vi "CodeKeithley.vi"(11 "SweepInfo":T1={"Current Range"=1e-10, "Source Measure Unit Channel (0: Channel A)"=0, "Waveform"={"t0"=timestamp(0 s since 1904-01-01), "dt"=1.0, "Y"=[]}, "VISA resource name"="", "CodeText"=""}) -> (0 "error out":errorcluster)   [LabVIEW 2020]
uses:
  Keithley 2600 Series/Keithley 2600 Series.lvlib
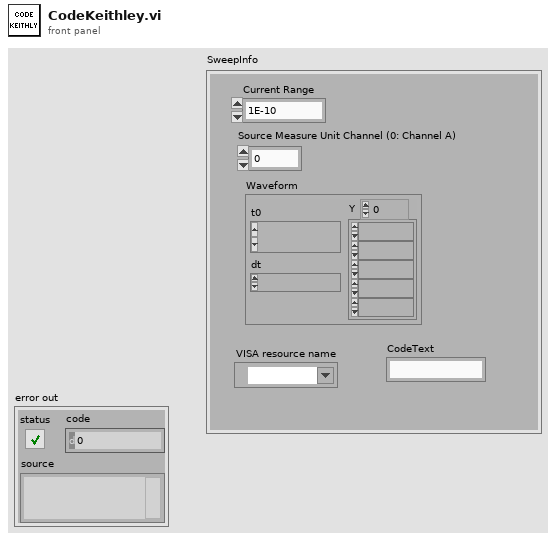
[diagram p1: front panel]
types:
  T1 = cluster{"Current Range":dbl, "Source Measure Unit Channel (0: Channel A)":i32, "Waveform":waveform(dbl), "VISA resource name":refnum<visa-resource-name>, "CodeText":string}
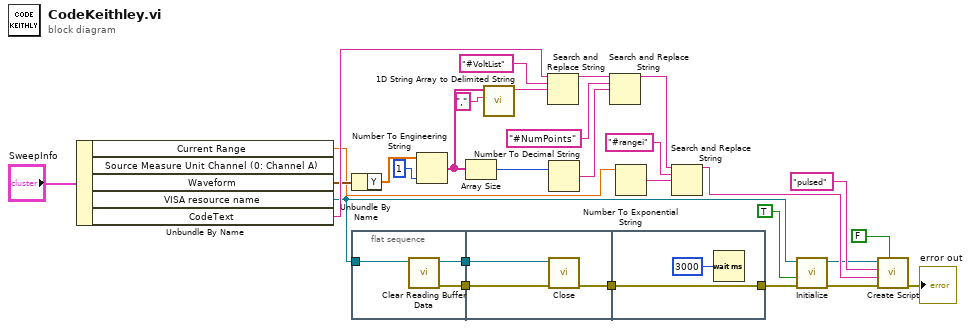
[diagram p0: block diagram]
diagram:
  n1 = Unbundle By Name("SweepInfo") -> ("Current Range"=w6:dbl, "Waveform"=w8:waveform(dbl), "VISA resource name"=w5:refnum<visa-resource-name>, "CodeText"=w9:string)  [unwired: 1 out]
  n2 = Unbundle By Name(w8) -> ("Y"=w20:dbl[])
  n3 = flat-sequence {
    tunnel: w5 -> [w32]
    tunnel: [w31] -> w4
    tunnel: [w30] -> w3
    tunnel: w4 -> [w35]
    tunnel: w3 -> [w34]
    tunnel: [w33] -> w2
    tunnel: [w36] -> w1
    tunnel: w2 -> [w36]
    frame #0 {
      n4 = call "Clear Reading Buffer Data.vi"("VISA resource name"=w32) -> ("error out"=w31:errorcluster, "VISA resource name out"=w30:refnum<visa-resource-name>)  [unwired: 9 in]
    }
    frame #1 {
      n5 = call "Close.vi"("error in (no error)"=w35, "VISA resource name"=w34) -> ("error out"=w33:errorcluster)  [unwired: 9 in]
    }
    frame #2 {
      n6 = Wait (ms)(milliseconds to wait=u32 3000) -> ()  [unwired: 1 out]
    }
  }
  n7 = Number To Engineering String(2:i16 1 ("precision (6)"), 4:w20) -> (0:w13:string[])  [unwired: 2 in]
  n8 = Array Size(array=w13) -> (size(s)=w12:i32)
  n9 = call <vilib>:"1D String Array to Delimited String.vi"("delimiter"=",", "string array"=w13) -> ("delimited string"=w15:string)  [unwired: 9 in]
  n10 = Search and Replace String(input string=w9, search string="#VoltList", replace string=w15) -> (result string=w14:string)  [unwired: 5 in, 3 out]
  n11 = Number To Decimal String(number=w12) -> (decimal integer string=w11:string)  [unwired: 1 in]
  n12 = Search and Replace String(input string=w14, search string="#NumPoints", replace string=w11) -> (result string=w27:string)  [unwired: 5 in, 3 out]
  n13 = Number To Exponential String(number=w6) -> (E-format string=w10:string)  [unwired: 3 in]
  n14 = Search and Replace String(input string=w27, search string="#rangei", replace string=w10) -> (result string=w28:string)  [unwired: 5 in, 3 out]
  n15 = call "Initialize.vi"("error in (no error)"=w1, "Reset (True)"=TRUE, "VISA resource name"=w5) -> ("error out"=w25:errorcluster, "VISA resource name out"=w22:refnum<visa-resource-name>)  [unwired: 7 in]
  n16 = call "Create Script.vi"("Auto Run (F: Disable)"=FALSE, "error in (no error)"=w25, "Source Code"=w28, "Script Variable"="pulsed", "VISA resource name"=w22) -> ("error out"=→"error out":errorcluster)  [unwired: 5 in, 1 out]
